vi "PratapLakeshore (SubVI).vi"(8 "error in (no error)":errorcluster, 9 "Channel":string, 10 "value to write":dbl, 11 "Instrument parameters in":T1) -> (0 "error out":errorcluster, 2 "Final temp":dbl, 3 "Instrument parameters out":T1)   [LabVIEW 2025]
uses:
  TYPE DEFS/S2DS_Instrument parameters.ctl
  Lake Shore 336.lvlib
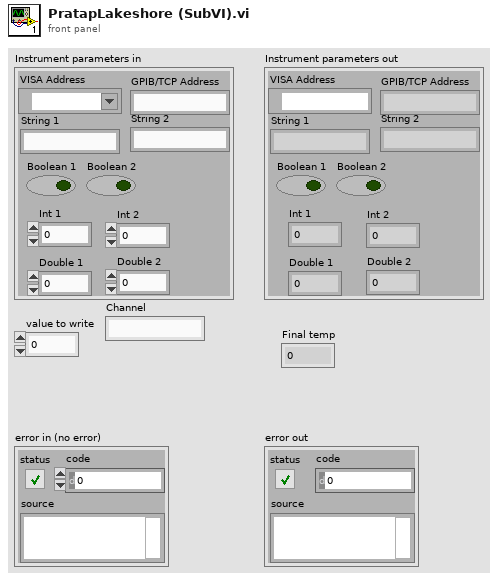
[diagram p1: front panel]
types:
  T1 = typedef "S2DS_Instrument parameters.ctl" = cluster{"VISA Address":refnum<visa-resource-name>, "GPIB/TCP Address":string, "String 1":string, "String 2":string, "Boolean 1":bool, "Boolean 2":bool, "Int 1":i32, "Int 2":i32, "Double 1":dbl, "Double 2":dbl}
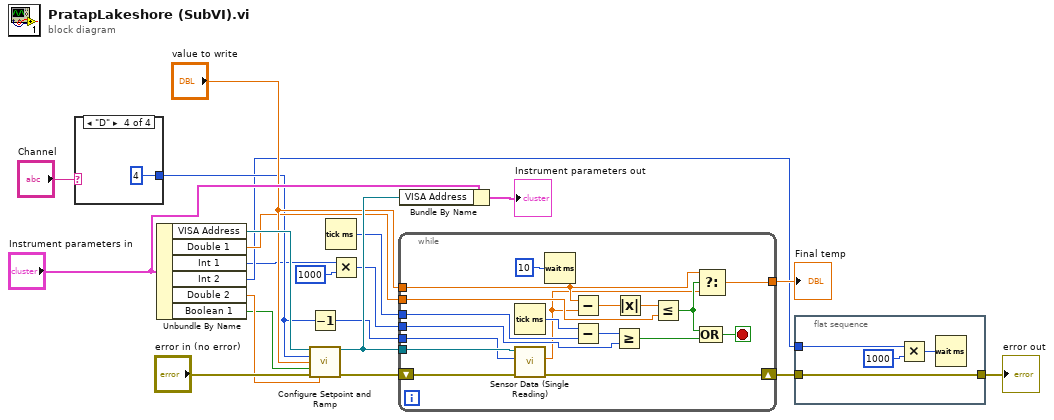
[diagram p0: block diagram]
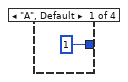
[diagram p2: hidden frame]
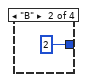
[diagram p3: hidden frame]
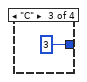
[diagram p4: hidden frame]
diagram:
  n1 = case shown="\"D\"" "Channel" {
    tunnel: [1 2 3 4] -> w5
    frame "A", Default {
    }
    frame "B" {
    }
    frame "C" {
    }
    frame "D" {
    }
  }
  n2 = Unbundle By Name("Instrument parameters in") -> ("VISA Address"=w18:refnum<visa-resource-name>, "Double 1"=w14:dbl, "Int 1"=w2:i32, "Int 2"=w4:i32, "Double 2"=w9:dbl, "Boolean 1"=w8:bool)
  n3 = Decrement(x=w5) -> (x-1=w7:i32)
  n4 = call "Configure Setpoint and Ramp.vi"("VISA resource name"=w18, "Output's Control Loop (1:1)"=w5, "Setpoint (0.00000)"="value to write", "Setpoint Ramping \nEnable (F: Off)"=w8, "error in (no error)"="error in (no error)", "Ramp Rate (0.0)"=w9) -> ("VISA resource name out"=w17:refnum<visa-resource-name>, "error out"=w16:errorcluster)  [unwired: 8 in]
  n5 = Tick Count (ms)() -> (millisecond timer value=w11:u32)
  n6 = Multiply(x=w2, y=1000) -> (x*y=w1:i32)
  n7 = while {
    tunnel: w17 -> [w43]
    shift-right: [w36] -> w13
    shift-left: w16 -> [w42]
    tunnel: "value to write" -> [w29]
    tunnel: w14 -> [w38]
    tunnel: w1 -> [w32]
    tunnel: w11 -> [w34]
    tunnel: [w27] -> w10
    tunnel: w7 -> [w26]
    stop <- w37 stop-if-true
    n8 = Tick Count (ms)() -> (millisecond timer value=w35:u32)
    n9 = call "Sensor Data (Single Reading).vi"("error in (no error)"=w42, "Input (0:A)"=w26, "VISA resource name"=w43) -> ("error out"=w36:errorcluster, "Sensor Data"=w28:dbl)  [unwired: 6 in, 1 out]
    n10 = Wait (ms)(milliseconds to wait=u32 10) -> ()  [unwired: 1 out]
    n11 = Subtract(x=w29, y=w28) -> (x-y=w40:dbl)
    n12 = Subtract(x=w35, y=w34) -> (x-y=w33:u32)
    n13 = Greater Or Equal?(x=w33, y=w32) -> (x >= y?=w31:bool)
    n14 = Absolute Value(x=w40) -> (abs(x)=w39:dbl)
    n15 = Less Or Equal?(x=w39, y=w38) -> (x <= y?=w30:bool)
    n16 = Select(t=w29, s=w30, f=w28) -> (s? t:f=w27:dbl)
    n17 = Compound Arithmetic op=OR(w30, w31) -> (w37:bool)
  }
  "Final temp" <- w10
  n18 = Bundle By Name(cluster="Instrument parameters in", "VISA Address"=w17) -> (→"Instrument parameters out":T1)
  n19 = flat-sequence {
    tunnel: w4 -> [w46]
    tunnel: w13 -> [w47]
    tunnel: [w47] -> w12
    frame #0 {
      n20 = Multiply(x=w46, y=1000) -> (x*y=w44:i32)
      n21 = Wait (ms)(milliseconds to wait=w44) -> ()  [unwired: 1 out]
    }
  }
  "error out" <- w12
